vi "VI Tree.vi"   [LabVIEW 2010, in "Stanford Research PS300 Series.lvlib"]
doc: "This is the instrument driver for the Stanford Research Systems PS 310/325/350 High Voltage Power Supplies. The VI Tree displays all the user-callable VIs of the instrument driver in an organized table.\n\nStanford Research Systems Series PS300\nCreated By: AC, NI,Austin, TX\nRelease Date: May, 1998\nOriginally Developed in LabVIEW Version: LabVIEW 4.1\n\nThis Instrument Driver's Revision number is: \"REV 1.0 , 01/1999, LV 4.1\" and is compatable with Instrument Firmware Revision: \"1.40\"."
uses:
  <instrlib>/Stanford Research PS300 Series/Stanford Research PS300 Series.lvlib
panel:
  # "© 2005 National Instruments.  ALL RIGHTS RESERVED."
  # "SEE DIAGRAM\nFOR VI TREE."
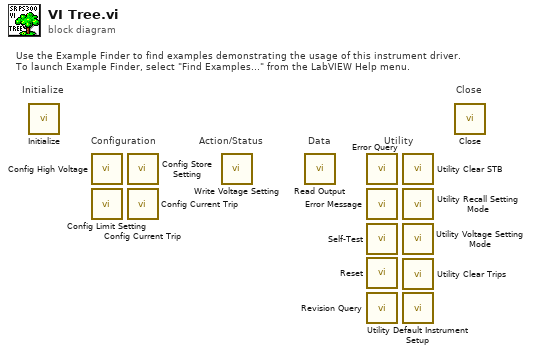
[diagram p0: block diagram]
diagram:
  # "Action/Status"
  # "Use the Example Finder to find examples demonstrating the usage of this instrument driver.\nTo launch Example Finder, select \"Find Examples...\" from the LabVIEW Help menu."
  # "Data"
  # "Configuration"
  # "Utility"
  # "Close"
  # "Initialize"
  n1 = call <instrlib>:"Initialize.vi"() -> ()  [unwired: 14 in, 2 out]
  n2 = call <instrlib>:"Config High Voltage.vi"() -> ()  [unwired: 14 in, 2 out]
  n3 = call <instrlib>:"Config Limit Setting.vi"() -> ()  [unwired: 14 in, 2 out]
  n4 = call <instrlib>:"Config Store Setting.vi"() -> ()  [unwired: 14 in, 2 out]
  n5 = call <instrlib>:"Config Current Trip.vi"() -> ()  [unwired: 14 in, 2 out]
  n6 = call <instrlib>:"Config Current Trip.vi"() -> ()  [unwired: 14 in, 2 out]
  n7 = call <instrlib>:"Write Voltage Setting.vi"() -> ()  [unwired: 14 in, 2 out]
  n8 = call <instrlib>:"Read Output.vi"() -> ()  [unwired: 13 in, 3 out]
  n9 = call <instrlib>:"Error Query.vi"() -> ()  [unwired: 12 in, 4 out]
  n10 = call <instrlib>:"Error Message.vi"() -> ()  [unwired: 11 in, 5 out]
  n11 = call <instrlib>:"Self-Test.vi"() -> ()  [unwired: 12 in, 4 out]
  n12 = call <instrlib>:"Reset.vi"() -> ()  [unwired: 14 in, 2 out]
  n13 = call <instrlib>:"Revision Query.vi"() -> ()  [unwired: 12 in, 4 out]
  n14 = call <instrlib>:"Utility Clear STB.vi"() -> ()  [unwired: 14 in, 2 out]
  n15 = call <instrlib>:"Utility Recall Setting Mode.vi"() -> ()  [unwired: 14 in, 2 out]
  n16 = call <instrlib>:"Utility Voltage Setting Mode.vi"() -> ()  [unwired: 13 in, 3 out]
  n17 = call <instrlib>:"Utility Clear Trips.vi"() -> ()  [unwired: 14 in, 2 out]
  n18 = call <instrlib>:"Utility Default Instrument Setup.vi"() -> ()  [unwired: 14 in, 2 out]
  n19 = call <instrlib>:"Close.vi"() -> ()  [unwired: 15 in, 1 out]
